vi "Read tactic_sequence.vi"(8 "error in (no error)":errorcluster, 11 "Role in":refnum<class "Role.lvclass">) -> (0 "error out":errorcluster, 2 "tactic_sequence":refnum<class "Tactic.lvclass">[](array[class]), 3 "Role out":refnum<class "Role.lvclass">)   [LabVIEW 2018, in "Role.lvclass"]
uses:
  Role.lvclass
  Tactic_class/Tactic.lvclass
  Role.lvclass/Role.ctl
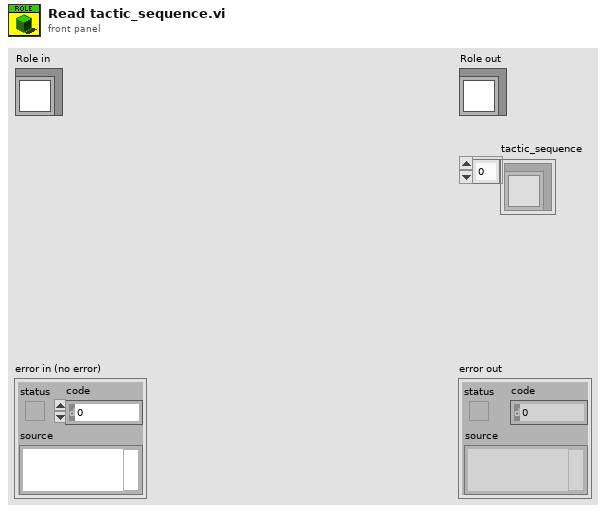
[diagram p1: front panel]
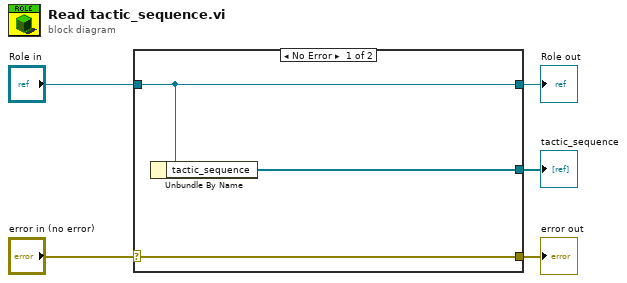
[diagram p0: block diagram]
diagram:
  n1 = case shown="No Error" "error in (no error)" {
    selector: "error in (no error)" -> [w8 w9]
    tunnel: [w8 w9] -> w4
    tunnel: [w7 w10] -> w2
    tunnel: "Role in" -> [w7 w10]
    tunnel: [w6 _] -> w1
    frame No Error {
      n2 = Unbundle By Name(w7) -> ("tactic_sequence"=w6:refnum<class "Tactic.lvclass">[])
    }
    frame Error {
    }
  }
  "error out" <- w4
  "Role out" <- w2
  "tactic_sequence" <- w1
